vi "LVPortInitEventStream.vi"(8 "error in":errorcluster, 10 "Category":string, 11 "ID":string) -> (0 "error out":errorcluster, 3 "Stream Info":T1)   [LabVIEW 2017]
uses:
  LVPortEventStreamType.ctl
  LVPortEventStreamDataType.ctl
  LVPortEventType.ctl
  LVPortEventRegistrationDataType.ctl
  LVPortEventGlobals.vi
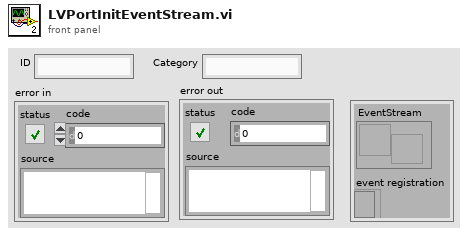
[diagram p1: front panel]
types:
  T1 = typedef "LVPortEventStreamType.ctl" = cluster{"EventStream":T2, "event registration":T3}
  T2 = typedef "LVPortEventStreamDataType.ctl" = refnum<user-event>
  T3 = typedef "LVPortEventRegistrationDataType.ctl" = refnum<event-registration>
  T4 = typedef "LVPortEventType.ctl" = cluster{"Name":string, "Data":variant}
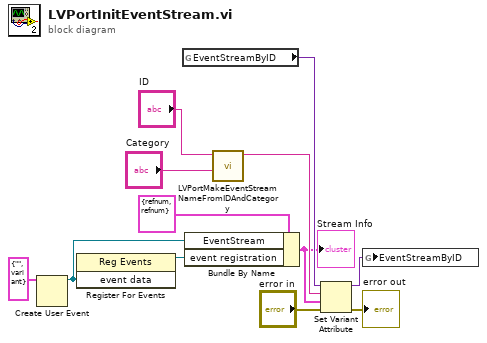
[diagram p0: block diagram]
diagram:
  n1 = Create User Event(user event datatype=T4 {"Name"="", "Data"=variant} ("event data")) -> (user event=w1:refnum<user-event>)  [unwired: 1 in, 1 out]
  n2 = register-events(w1) -> (reference out=w4:refnum<event-registration>)  [unwired: 2 in, 1 out]
  n3 = global read "LVPortEventGlobals.vi" "EventStreamByID"() -> (w10:variant)
  n4 = Bundle By Name(cluster=T1 {"EventStream"=refnum, "event registration"=refnum} ("EventStreamInfo"), "EventStream"=w1, "event registration"=w4) -> (w3:T1)
  "Stream Info" <- w3
  n5 = call "LVPortMakeEventStreamNameFromIDAndCategory.vi"("Category"="Category", "ID"="ID") -> ("StreamName"=w8:string)  [unwired: 9 in]
  n6 = Set Variant Attribute(Variant=w10, name=w8, value=w3, error in="error in") -> (Variant out=w9:variant, error out=→"error out":errorcluster)  [unwired: 1 out]
  n7 = global write "LVPortEventGlobals.vi" "EventStreamByID"(w9) -> ()
